vi "Add Items to ListView by Text Array.vi"(8 "error in (no error)":errorcluster caption="错误输入（无错误）", 10 "Text":string[](array[string]), 11 "ListViewClass 输入":refnum<class "ListViewClass.lvclass"> caption="DNL_LabVIEW Object in") -> (0 "error out":errorcluster caption="错误输出", 3 "ListViewClass 输出":refnum<class "ListViewClass.lvclass"> caption="DNL_LabVIEW Object out")   [LabVIEW 2012, in "ListViewClass.lvclass"]
uses:
  ListViewClass.lvclass
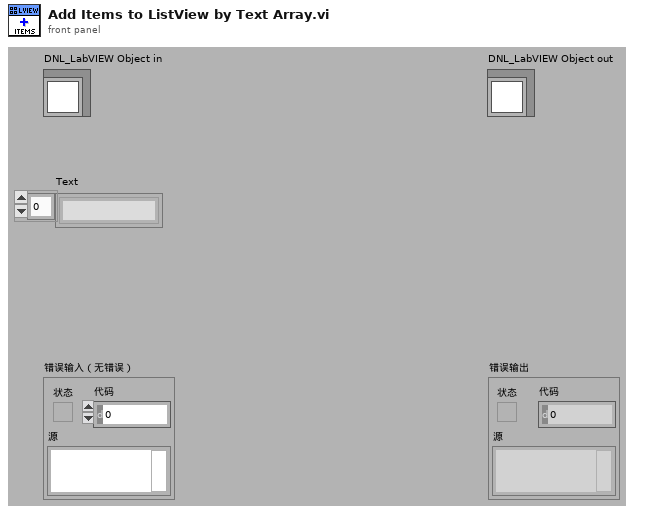
[diagram p1: front panel]
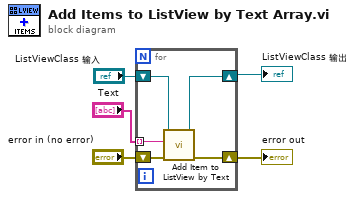
[diagram p0: block diagram]
diagram:
  n1 = for {
    shift-right: [w9] -> w4
    shift-left: "ListViewClass 输入" -> [w10]
    shift-right: [w8] -> w2
    shift-left: "error in (no error)" -> [w7]
    tunnel: "Text" -> [w6] mode=indexing
    n2 = call "Add Item to ListView by Text.vi"("error in (no error)"=w7, "Text"=w6, "ListViewClass 输入"=w10) -> ("error out"=w8:errorcluster, "ListViewClass 输出"=w9:refnum<class "ListViewClass.lvclass">)  [unwired: 7 in]
  }
  "error out" <- w2
  "ListViewClass 输出" <- w4
